vi "Prepare Glue.vi"(7 "Console Log in":refnum<class "Console Log.lvclass">, 8 "error in":errorcluster, 11 "Gluing Procedure in":refnum<class "Gluing Procedure.lvclass">) -> (0 "error out":errorcluster, 1 "Step canceled?":bool, 3 "Gluing Procedure out":refnum<class "Gluing Procedure.lvclass">, 5 "Console Log out":refnum<class "Console Log.lvclass">)   [LabVIEW 2011]
uses:
  Procedure Classes/Gluing Procedure/Gluing Procedure.lvclass
  Potting Application/UI Classes/Console Log/Console Log.lvclass
panel:
  in  "Cancel Button":bool
  in  "OK Button":bool
  in  "time stamp":timestamp
  # "Prepare Glue!"
  # "This VI simply prompts the user to prepare the glue before operation of the main gluing motion"
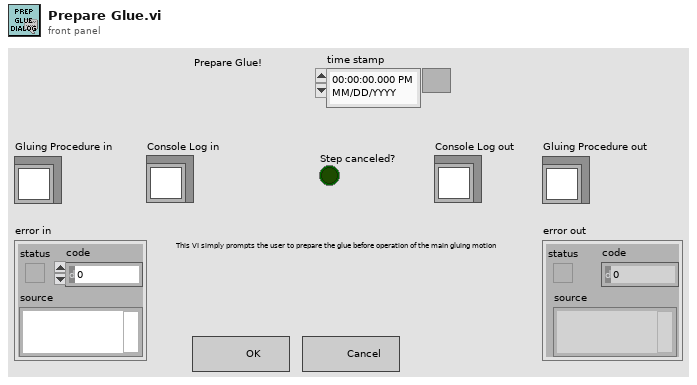
[diagram p1: front panel]
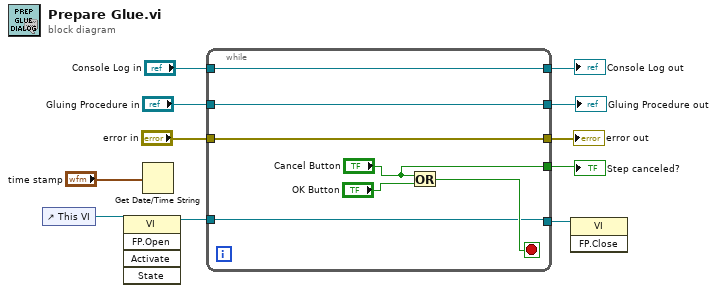
[diagram p0: block diagram]
diagram:
  n1 = control-ref of="This VI"() -> (w3:refnum<vi>)
  n2 = invoke class="VI" method="FP.Open"(reference=w3) -> (reference out=w2:refnum<vi>)  [unwired: 4 in, 4 out]
  n3 = Get Date/Time String(seconds (now)="time stamp") -> ()  [unwired: 2 in, 2 out]
  n4 = while {
    tunnel: ["Cancel Button"] -> w10
    tunnel: "Console Log in" -> [w15]
    tunnel: [w15] -> w8
    tunnel: "Gluing Procedure in" -> [w14]
    tunnel: [w14] -> w6
    tunnel: "error in" -> [w13]
    tunnel: [w13] -> w4
    tunnel: w2 -> [w12]
    tunnel: [w12] -> w1
    stop <- w16 stop-if-true
    n5 = Or(x="Cancel Button", y="OK Button") -> (x .or. y?=w16:bool)
  }
  "error out" <- w4
  "Gluing Procedure out" <- w6
  "Console Log out" <- w8
  "Step canceled?" <- w10
  n6 = invoke class="VI" method="FP.Close"(reference=w1) -> ()  [unwired: 2 in, 3 out]
